vi "Restore Configuration.vi"(8 "error in (no error)":errorcluster, 10 "File path":path, 11 "Measure Object in":refnum<class "Application Controller.lvclass">) -> (0 "error out":errorcluster, 1 "Section out":string, 2 "File path out":path, 3 "Measure Object out":refnum<class "Application Controller.lvclass">)   [LabVIEW 2016, in "Application Controller.lvclass"]
uses:
  Application Controller.lvclass
  Application Controller.lvclass/Application Controller.ctl
  Read Monitor ref.vi
  NHMFL_Core/Libraries/Queued Listbox/Queued Listbox.xctl
  Process Controller/Process Controller.lvclass
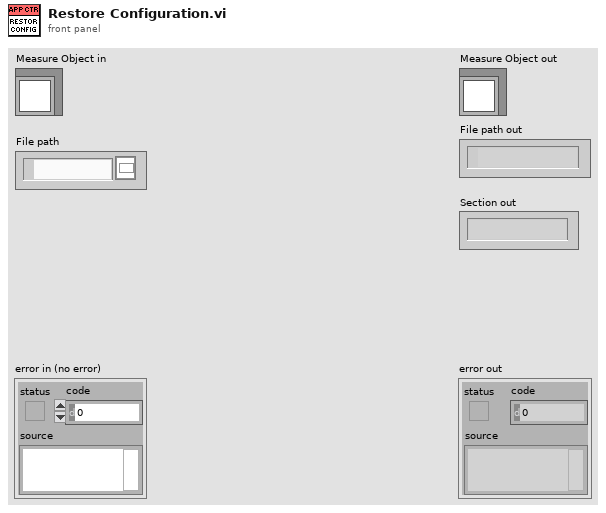
[diagram p1: front panel]
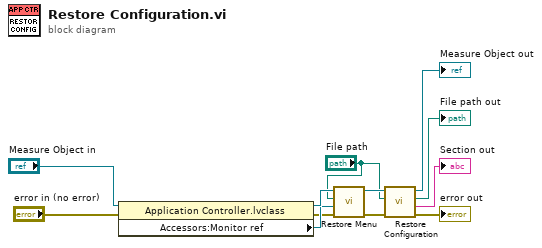
[diagram p0: block diagram]
diagram:
  n1 = property class="Application Controller.lvclass"(reference="Measure Object in", error in="error in (no error)") -> (reference out=w8:refnum<class "Application Controller.lvclass">, error out=w3:errorcluster, "Accessors:Monitor ref"=w7:refnum<vi>)
  n2 = call-dynamic "Restore Menu.vi"("error in (no error)"=w3, "Menu ref"=w7, "File path"="File path", "Monitor-Pulse in"=w8) -> ("error out"=w2:errorcluster, "Monitor-Pulse out"=w5:refnum<class "Application Controller.lvclass">)  [unwired: 4 in, 2 out]
  n3 = call-parent "Restore Configuration.vi"("error in (no error)"=w2, "File path"="File path", "Measure Object in"=w5) -> ("error out"=→"error out":errorcluster, "Section out"=→"Section out":string, "File path out"=→"File path out":path, "Measure Object out"=→"Measure Object out":refnum<class "Application Controller.lvclass">)  [unwired: 5 in]
